vi "INTELLIFAUCET Temp Adjustment.vi"(0 "VISA session":refnum<visa-resource-name>="MW100", 1 "Target":dbl=58.0, 3 "Reading":dbl=57.8, 4 "K(0.1)":dbl=0.1, 5 "Error In":errorcluster, 6 "TEMP,FLOW":T3=enum."FLOW", 7 "Debug":bool, 8 "Elapsed Time (sec)":dbl, 9 "State":T1, 10 "PID gains":T4={"proportional gain (Kc)"=0.1, "integral time (Ti, min)"=0.01, "derivative time (Td, min)"=0.0} {"derivative time (Td, min)" format="%.3f"; "integral time (Ti, min)" format="%.3f"; "proportional gain (Kc)" format="%.3f"}, 11 "Refnum in":T2, 12 "output range":cluster{"output high":dbl, "output low":dbl}={"output high"=140.0, "output low"=40.0} {"output low" format="%.2f"; "output high" format="%.2f"}, 13 "Use Fuzzy Logic":bool, 17 "Use Proportion Valve":bool, 18 "ErrorPassBand(%)":dbl=0.01) -> (14 "VISA session out":refnum<visa-resource-name>="MW100", 15 "Intellif Valve % Open":dbl, 16 "uA Output":i32, 19 "Error Out":errorcluster)   [LabVIEW 2016]
uses:
  Type Definitions/INTELLIFAUCT Temp Flow.ctl
  Type Definitions/HEWH Purge Draw.ctl
  Type Definitions/INTELLIFAUCET Set Mode.ctl
panel:
  out "Adjustment Factor":dbl
  out "Control Variable (Temp/GPM) Output":dbl=59.99100089774931 format="%.2f"
  out "Going into Correction Loop?":bool=TRUE
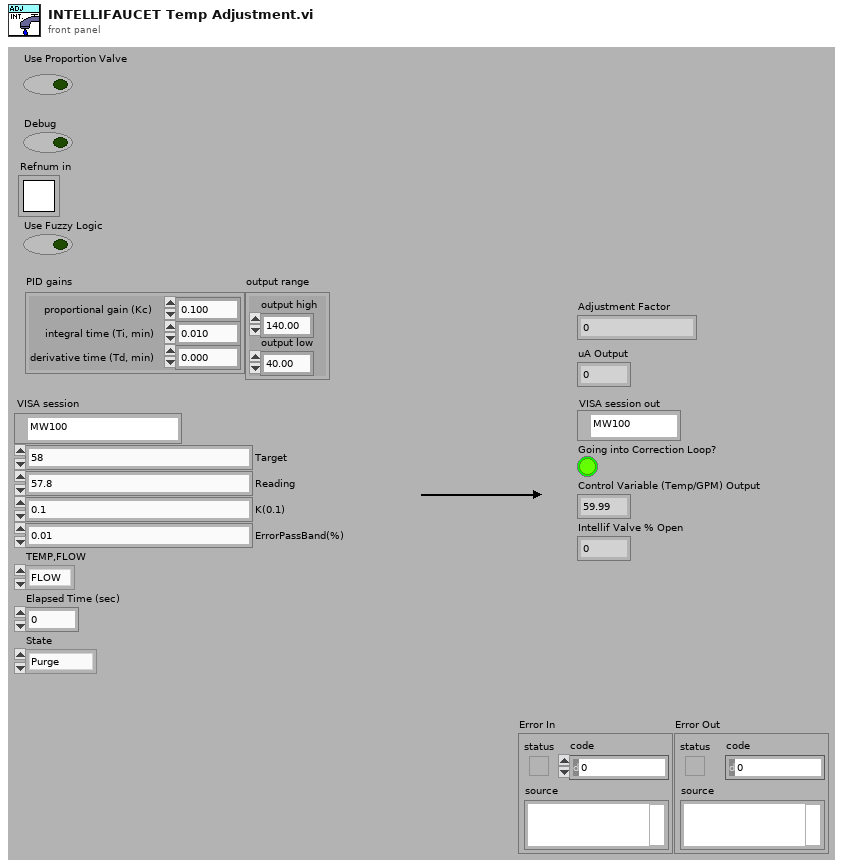
[diagram p1: front panel]
types:
  T1 = typedef "HEWH Purge Draw.ctl" = enum16{"Purge", "Draw"}
  T2 = typedef "Semaphore RefNum" = refnum<k1>
  T3 = typedef "INTELLIFAUCT Temp Flow.ctl" = enum8{"TEMP", "FLOW"}
  T4 = cluster{"proportional gain (Kc)":dbl, "integral time (Ti, min)":dbl, "derivative time (Td, min)":dbl}
  T5 = typedef "INTELLIFAUCET Set Mode.ctl" = enum16{"Adjust Temp", "Adjust Flow", "Start Flow", "Stop Flow", "Hold"}
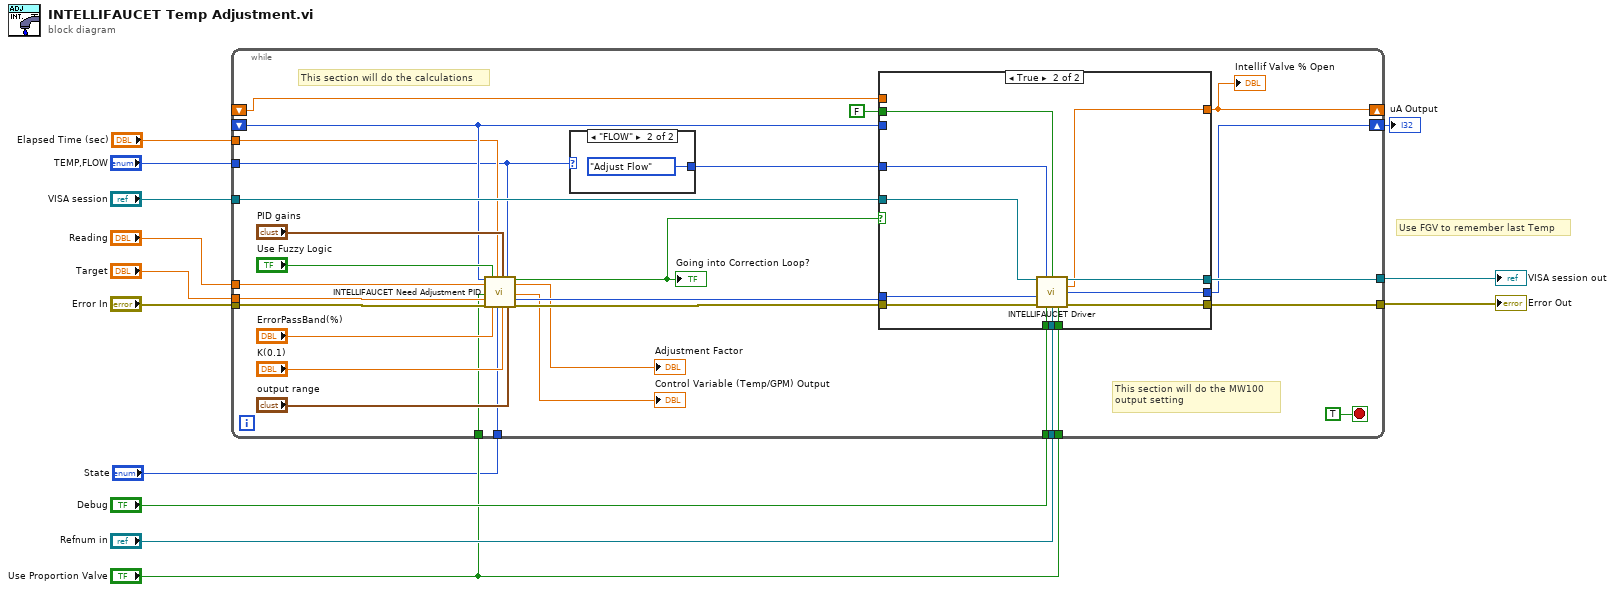
[diagram p0: block diagram]
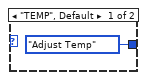
[diagram p2: hidden frame]
diagram:
  # "Use FGV to remember last Temp"
  n1 = while {
    tunnel: "VISA session" -> [w42]
    tunnel: "Error In" -> [w38]
    tunnel: [w41] -> w11
    tunnel: "Reading" -> [w29]
    tunnel: "Target" -> [w39]
    tunnel: [w40] -> w8
    tunnel: "TEMP,FLOW" -> [w14]
    tunnel: "Debug" -> [w31]
    tunnel: "Refnum in" -> [w30]
    shift-right: [w28] -> w3
    shift-left: _ -> [w20]
    shift-right: [w22] -> _
    shift-left: _ -> [w21]
    tunnel: "Use Proportion Valve" -> [w19]
    tunnel: "Use Proportion Valve" -> [w18]
    tunnel: "State" -> [w16]
    tunnel: "Elapsed Time (sec)" -> [w15]
    stop <- TRUE stop-if-true
    # "This section will do the MW100\noutput setting"
    # "This section will do the calculations"
    n2 = call "INTELLIFAUCET Need Adjustment PID.vi"("Previous MicroAmp"=w20, "GPM reading"=w29, "Use Proportion Valve"=w18, "GPM Target(3)"=w39, "Error In"=w38, "Use Fuzzy Logic"="Use Fuzzy Logic", "ErrorPassBand(%)"="ErrorPassBand(%)", "Elapsed Time (sec)"=w15, "State"=w16, "PID gains"="PID gains", "K(0.1)"="K(0.1)", "TEMP,FLOW"=w14, "output range"="output range") -> ("Going into Correction Loop?"=w36:bool, "Adjustment Factor"=→"Adjustment Factor":dbl, "Control Variable (Temp/GPM) Output"=→"Control Variable (Temp/GPM) Output":dbl, "Micro Amp"=w25:i32, "Error Out"=w37:errorcluster)  [unwired: 2 in]
    "Going into Correction Loop?" <- w36
    n3 = case shown="\"FLOW\"" w14 {
      tunnel: [INTELLIFAUCET_Set_Mode."Adjust Temp" ("Mode") INTELLIFAUCET_Set_Mode."Adjust Flow" ("Mode")] -> w26
      frame "TEMP", Default {
      }
      frame "FLOW" {
      }
    }
    n4 = case shown="False" w36 {
      tunnel: w42 -> [w48 w61]
      tunnel: w37 -> [w49 w60]
      tunnel: [w49 w59] -> w41
      tunnel: [w48 w58] -> w40
      tunnel: w31 -> [_ w57]
      tunnel: w30 -> [_ w56]
      tunnel: [w47 w55] -> w28
      tunnel: w20 -> [w47 _]
      tunnel: w26 -> [_ w54]
      tunnel: FALSE ("Use General Conversion") -> [_ w53]
      tunnel: w25 -> [_ w51]
      tunnel: [w46 w52] -> w22
      tunnel: w21 -> [w46 _]
      tunnel: w19 -> [_ w50]
      frame False {
      }
      frame True {
        n5 = call "INTELLIFAUCET Driver.vi"("VISA session"=w61, "Mode"=w54, "Use General Conversion"=w53, "uA Set"=w51, "Error In"=w60, "Debug"=w57, "Refnum in"=w56, "Use Proportion Valve"=w50) -> ("VISA session out"=w58:refnum<visa-resource-name>, "Intellif Valve % Open"=w52:dbl, "uA Output"=w55:i32, "Error Out"=w59:errorcluster)  [unwired: 4 in]
      }
    }
    "Intellif Valve % Open" <- w22
  }
  "Error Out" <- w11
  "VISA session out" <- w8
  "uA Output" <- w3
